vi "DSF.Engine.Framework.Get All Transfer Groups.vi"(11 "Framework in":refnum<class "DSF.Engine.Framework.lvclass">) -> (2 "All Transfer Groups":refnum<class "DSF.Engine.Transfer Group.lvclass">[](array[class]), 3 "Framework out":refnum<class "DSF.Engine.Framework.lvclass">)   [LabVIEW 2017, in "Data Sharing Framework Engine.lvlib" / "DSF.Engine.Framework.lvclass"]
uses:
  DSF.Engine.Framework.lvclass
  Transfer/DSF.Engine.Transfer Group.lvclass
  DSF.Engine.Framework.lvclass/DSF.Engine.Framework.ctl
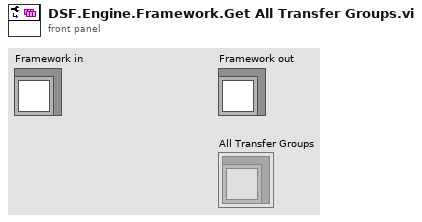
[diagram p1: front panel]
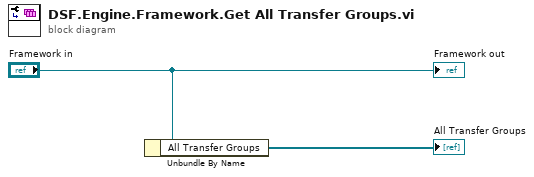
[diagram p0: block diagram]
diagram:
  n1 = Unbundle By Name("Framework in") -> ("All Transfer Groups"=→"All Transfer Groups":refnum<class "DSF.Engine.Transfer Group.lvclass">[])
  "Framework out" <- "Framework in"
